vi "11102 UI.vi"(8 "error in (no error)":errorcluster, 11 "Node Ptr":T1 format="%.0x") -> (0 "error out":errorcluster)   [LabVIEW 2016, in "Modules.lvlib" / "11102.lvclass"]
uses:
  11102.lvclass
  <vilib>/NI Veristand/Custom Device API/Custom Device Item Ref.ctl
  RSI Module/SubPanel Command.ctl
  C:/git-external/Scan-Engine-Custom-Device-Classes/Source/RemIO Module/RemIO Module.lvclass
  11102.lvclass/11102.ctl
  <vilib>/indcomecat/Remote IO/typedefs/REM-11102/channul number REM-11102.ctl
  RemIO Module/RemIO Module.lvclass
  <vilib>/indcomecat/Remote IO/NI ECAT Remote IO.lvlib
  <vilib>/NI Veristand/Custom Device API/Custom Device API.lvlib
  RSI Module/RSI Module.lvclass
panel:
  in  "Mean Value 3":u8(ring) items=["16-sample", "no mean-value", "4-sample", "32-sample"]
  in  "Mean Value 2":u8(ring) items=["16-sample", "no mean-value", "4-sample", "32-sample"]
  in  "Mean Value 1":u8(ring) items=["16-sample", "no mean-value", "4-sample", "32-sample"]
  in  "Input Filter 3":u8(ring) items=["30 Hz", "12 kHz"]
  in  "Input Filter 2":u8(ring) items=["30 Hz", "12 kHz"]
  in  "Input Filter 1":u8(ring) items=["30 Hz", "12 kHz"]
  in  "Input Range 3":u8(ring) items=["0 mA ... 20 mA"=4, "-20 mA ... 20 mA"=5, "4 mA ... 20 mA"=6, "Channel inactive"=15]
  in  "Input Range 2":u8(ring) items=["0 mA ... 20 mA"=4, "-20 mA ... 20 mA"=5, "4 mA ... 20 mA"=6, "Channel inactive"=15]
  in  "Input Range 1":u8(ring) items=["0 mA ... 20 mA"=4, "-20 mA ... 20 mA"=5, "4 mA ... 20 mA"=6, "Channel inactive"=15]
  out "_MeanVallabel":string="Mean-Value"
  in  "Mean Value 0":u8(ring) items=["16-sample", "no mean-value", "4-sample", "32-sample"]
  out "_InFilterlabel":string="Input Filter Time"
  in  "Input Filter 0":u8(ring) items=["30 Hz", "12 kHz"]
  out "_Chan0Label":string="Channel 0"
  out "_Chan1Label":string="Channel 1"
  out "_Chan2Label":string="Channel 2"
  out "_Chan3Label":string="Channel 3"
  out "_Rangelabel":string="Measuring Range"
  in  "Input Range 0":u8(ring) items=["0 mA ... 20 mA"=4, "-20 mA ... 20 mA"=5, "4 mA ... 20 mA"=6, "Channel inactive"=15]
  in  "SubPanel Event":refnum<user-event>
  in  "Header":cluster{"Section Name":string}={"Section Name"="NI REM-11102 Settings"}
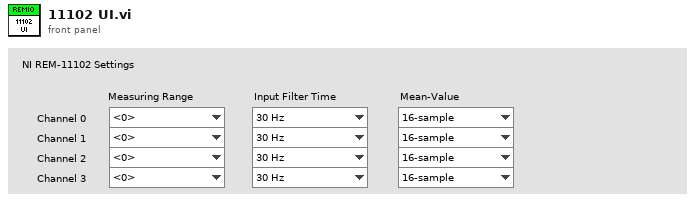
[diagram p1: front panel]
types:
  T1 = typedef "Custom Device API.lvlib/Custom Device Item Ref.ctl" = u64
  T2 = typedef "NI ECAT Remote IO.lvlib/channul number REM-11102.ctl" = u8
  T3 = typedef "NI ECAT Remote IO.lvlib/input filter time REM-11102.ctl" = u8
  T4 = typedef "NI ECAT Remote IO.lvlib/mean-value REM-11102.ctl" = u8
  T5 = typedef "NI ECAT Remote IO.lvlib/measuring range REM-11102.ctl" = u8
  T6 = cluster{"channel number":T2, "input filter time":T3, "mean-value":T4, "measuring range":T5}[]
  T7 = cluster{"channel number":T2, "input filter time":T3, "mean-value":T4, "measuring range":T5}
  T8 = typedef "Modules.lvlib/RSI Module.lvclass/SubPanel Command.ctl" = enum16{"Stop"}
  T9 = cluster{"channel number":T2, "Input Filter 0":u8, "Mean Value 0":u8, "Input Range 0":u8}
  T10 = cluster{"channel number":T2, "Input Filter 1":u8, "Mean Value 1":u8, "Input Range 1":u8}
  T11 = cluster{"channel number":T2, "Input Filter 2":u8, "Mean Value 2":u8, "Input Range 2":u8}
  T12 = cluster{"channel number":T2, "Input Filter 3":u8, "Mean Value 3":u8, "Input Range 3":u8}
  T13 = cluster{"channel number":T2, "Input Filter 3":u8, "Mean Value 3":u8, "Input Range 3":u8}[]
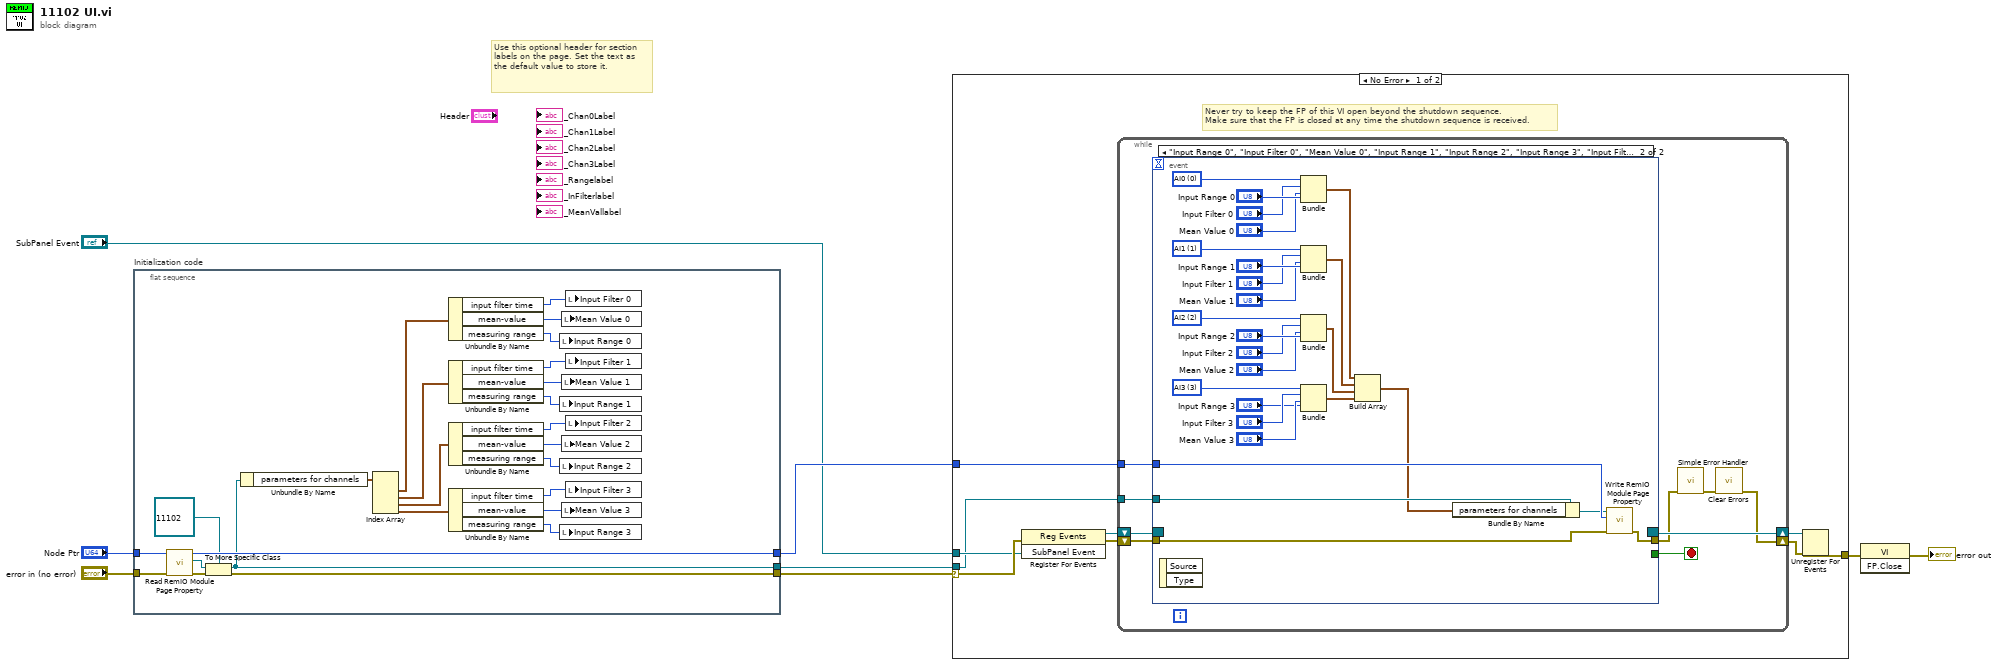
[diagram p0: block diagram]
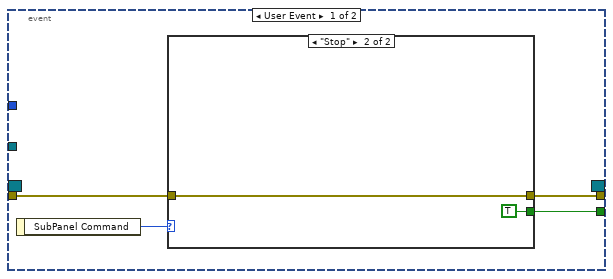
[diagram p2: hidden frame]
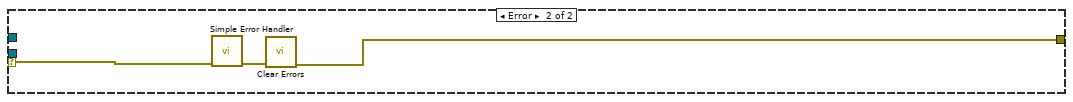
[diagram p4: hidden frame]
diagram:
  # "Use this optional header for section labels on the page. Set the text as the default value to store it."
  n1 = flat-sequence "Initialization code" {
    tunnel: "error in (no error)" -> [w32]
    tunnel: "Node Ptr" -> [w33]
    tunnel: [w28] -> w2
    tunnel: [w31] -> w5
    tunnel: [w26] -> w1
    frame #0 {
      n2 = call "Read RemIO Module Page Property.vi"("error in (no error)"=w32, "Node Ptr In"=w33) -> ("error out"=w30:errorcluster, "RemIO Module"=w29:refnum<class "RemIO Module.lvclass">, "Node Ptr Out"=w31:T1)  [unwired: 7 in]
      n3 = To More Specific Class(target class=refnum<class "11102.lvclass"> refnum ("Modules.lvlib:11102.lvclass"), reference=w29, error in=w30) -> (specific class reference=w26:refnum<class "11102.lvclass">, error out=w28:errorcluster)
      n4 = Unbundle By Name(w26) -> ("parameters for channels"=w12:T6)
      n5 = Index Array(array=w12) -> (element #1=w25:T7, element #2=w11:T7, element #3=w10:T7, element #4=w9:T7)  [unwired: 4 in]
      n6 = Unbundle By Name(w25) -> ("input filter time"=w22:T3, "mean-value"=w24:T4, "measuring range"=w23:T5)
      n7 = Unbundle By Name(w11) -> ("input filter time"=w21:T3, "mean-value"=w19:T4, "measuring range"=w20:T5)
      n8 = Unbundle By Name(w10) -> ("input filter time"=w16:T3, "mean-value"=w18:T4, "measuring range"=w17:T5)
      n9 = Unbundle By Name(w9) -> ("input filter time"=w15:T3, "mean-value"=w13:T4, "measuring range"=w14:T5)
      n10 = local write "Input Range 0"(w23) -> ()
      n11 = local write "Input Range 1"(w20) -> ()
      n12 = local write "Input Range 2"(w17) -> ()
      n13 = local write "Input Range 3"(w14) -> ()
      n14 = local write "Mean Value 0"(w24) -> ()
      n15 = local write "Mean Value 1"(w19) -> ()
      n16 = local write "Mean Value 2"(w18) -> ()
      n17 = local write "Mean Value 3"(w13) -> ()
      n18 = local write "Input Filter 0"(w22) -> ()
      n19 = local write "Input Filter 1"(w21) -> ()
      n20 = local write "Input Filter 2"(w16) -> ()
      n21 = local write "Input Filter 3"(w15) -> ()
    }
  }
  n22 = case shown="No Error" w2 {
    selector: w2 -> [w36 w87]
    tunnel: [w40 w85] -> w8
    tunnel: w5 -> [w37 _]
    tunnel: "SubPanel Event" -> [w35 _]
    tunnel: w1 -> [w34 _]
    frame No Error {
      # "Never try to keep the FP of this VI open beyond the shutdown sequence.\nMake sure that the FP is closed at any time the shutdown sequence is received."
      n23 = register-events(error in=w36, w35) -> (reference out=w38:refnum<event-registration>, error out=w39:errorcluster)  [unwired: 1 in]
      n24 = while {
        tunnel: w37 -> [w47]
        shift-right: [w44] -> w41
        shift-left: w39 -> [w50]
        shift-right: [w51] -> w42
        shift-left: w38 -> [w49]
        tunnel: w34 -> [w43]
        stop <- w48 stop-if-true
        n25 = event shown="[1] \"Input Range 0\", \"Input Filter 0\", \"Mean Value 0\", \"Input Range 1\", \"Input Range 2\", \"Input Range 3\", \"Input Filter 1\", \"Input Filter 2\", \"Input Filter 3\", \"Mean Value 1\", \"Mean Value 2\", \"Mean Value 3\": Value Change" {
          selector: w49 -> [_ _]
          dyn-events: [_ _] -> w51
          timeout: _ -> [_ _]
          tunnel: w50 -> [w54 w82]
          tunnel: [w52 _] -> w48
          tunnel: [w53 w81] -> w46
          tunnel: w47 -> [_ w83]
          tunnel: w43 -> [_ w84]
          event User Event {
            n26 = event-data() -> ("SubPanel Command"=w55:T8)  [unwired: 1 out]
            n27 = case shown="\"Stop\"" w55 {
              tunnel: w54 -> [w56 w57]
              tunnel: [w56 w57] -> w53
              tunnel: [_ TRUE] -> w52
              frame Default {
              }
              frame "Stop" {
              }
            }
          }
          event "Input Range 0", "Input Filter 0", "Mean Value 0", "Input Range 1", "Input Range 2", "Input Range 3", "Input Filter 1", "Input Filter 2", "Input Filter 3", "Mean Value 1", "Mean Value 2", "Mean Value 3": Value Change {
            w73 = T2 3 items=["AI0", "AI1", "AI2", "AI3"] ("channel number")
            w72 = T2 2 items=["AI0", "AI1", "AI2", "AI3"] ("channel number")
            w76 = T2 1 items=["AI0", "AI1", "AI2", "AI3"] ("channel number")
            w77 = T2 0 items=["AI0", "AI1", "AI2", "AI3"] ("channel number")
            n28 = event-data() -> ()  [unwired: 3 out]
            n29 = Bundle("channel number"=w77, "Input Filter 0"="Input Filter 0", "Mean Value 0"="Mean Value 0", "Input Range 0"="Input Range 0") -> (w79:T9)  [unwired: 1 in]
            n30 = Bundle("channel number"=w76, "Input Filter 1"="Input Filter 1", "Mean Value 1"="Mean Value 1", "Input Range 1"="Input Range 1") -> (w78:T10)  [unwired: 1 in]
            n31 = Bundle("channel number"=w72, "Input Filter 2"="Input Filter 2", "Mean Value 2"="Mean Value 2", "Input Range 2"="Input Range 2") -> (w60:T11)  [unwired: 1 in]
            n32 = Bundle("channel number"=w73, "Input Filter 3"="Input Filter 3", "Mean Value 3"="Mean Value 3", "Input Range 3"="Input Range 3") -> (w61:T12)  [unwired: 1 in]
            n33 = Build Array(w79, w78, w60, w61) -> (w59:T13)
            n34 = Bundle By Name(cluster=w84, "parameters for channels"=w59) -> (w80:refnum<class "11102.lvclass">)
            n35 = call "Write RemIO Module Page Property.vi"("error in (no error)"=w82, "Node Ptr In"=w83, "RemIO Module"=w80) -> ("error out"=w81:errorcluster)  [unwired: 6 in, 2 out]
          }
        }
        n36 = call <vilib>:"Simple Error Handler.vi"("error in (no error)"=w46) -> ("error out"=w45:errorcluster)  [unwired: 1 in, 7 out]
        n37 = call <vilib>:"Clear Errors.vi"("error in (no error)"=w45) -> ("error out"=w44:errorcluster)  [unwired: 1 in, 5 out]
      }
      n38 = Unregister For Events(event registration refnum=w42, error in=w41) -> (error out=w40:errorcluster)
    }
    frame Error {
      n39 = call <vilib>:"Simple Error Handler.vi"("error in (no error)"=w87) -> ("error out"=w86:errorcluster)  [unwired: 1 in, 7 out]
      n40 = call <vilib>:"Clear Errors.vi"("error in (no error)"=w86) -> ("error out"=w85:errorcluster)  [unwired: 1 in, 5 out]
    }
  }
  n41 = invoke class="VI" method="FP.Close"(error in=w8) -> (error out=→"error out":errorcluster)  [unwired: 2 in, 2 out]
